vi "Read Diagrams.vi"(9 "Structure in":refnum<class "Structure.lvclass">) -> (3 "Structure out":refnum<class "Structure.lvclass">, 4 "Diagrams":refnum<class "Diagram.lvclass">[](array[class]))   [LabVIEW 2014, in "Raspberry Pi Compatible Compiler for LabVIEW.lvlib" / "Structure.lvclass"]
uses:
  Structure.lvclass
  Diagram/Diagram.lvclass
  Structure.lvclass/Structure.ctl
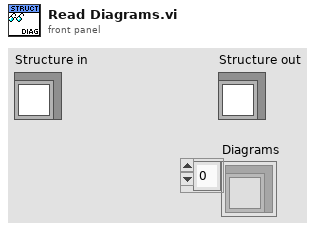
[diagram p1: front panel]
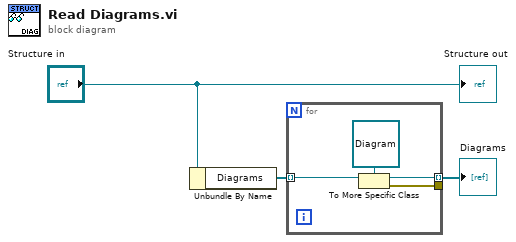
[diagram p0: block diagram]
diagram:
  n1 = Unbundle By Name("Structure in") -> ("Diagrams"=w2:refnum<class "GObject.lvclass">[])
  n2 = for {
    tunnel: w2 -> [w7] mode=indexing
    tunnel: [w6] -> w1 mode=indexing
    tunnel: [w4] -> _
    n3 = To More Specific Class(target class=refnum<class "Diagram.lvclass"> refnum ("Diagram.lvclass"), reference=w7) -> (specific class reference=w6:refnum<class "Diagram.lvclass">, error out=w4:errorcluster)  [unwired: 1 in]
  }
  "Diagrams" <- w1
  "Structure out" <- "Structure in"
